vi "operate.vi"(10 "symbol":string[](array[string]), 11 "Element":string[](array[string])) -> (2 "Value":dbl, 3 "Result":string)   [LabVIEW 2020]
uses:
  <vilib>/Analysis/NI_AALBase.lvlib
  <vilib>/Analysis/baseanly.llb/Mean (DBL).vi
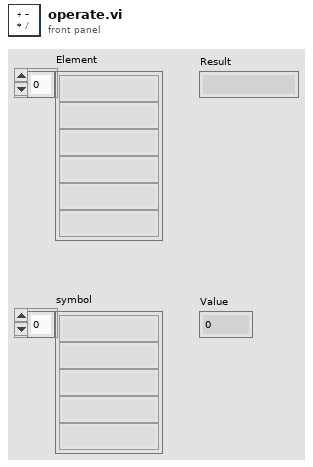
[diagram p1: front panel]
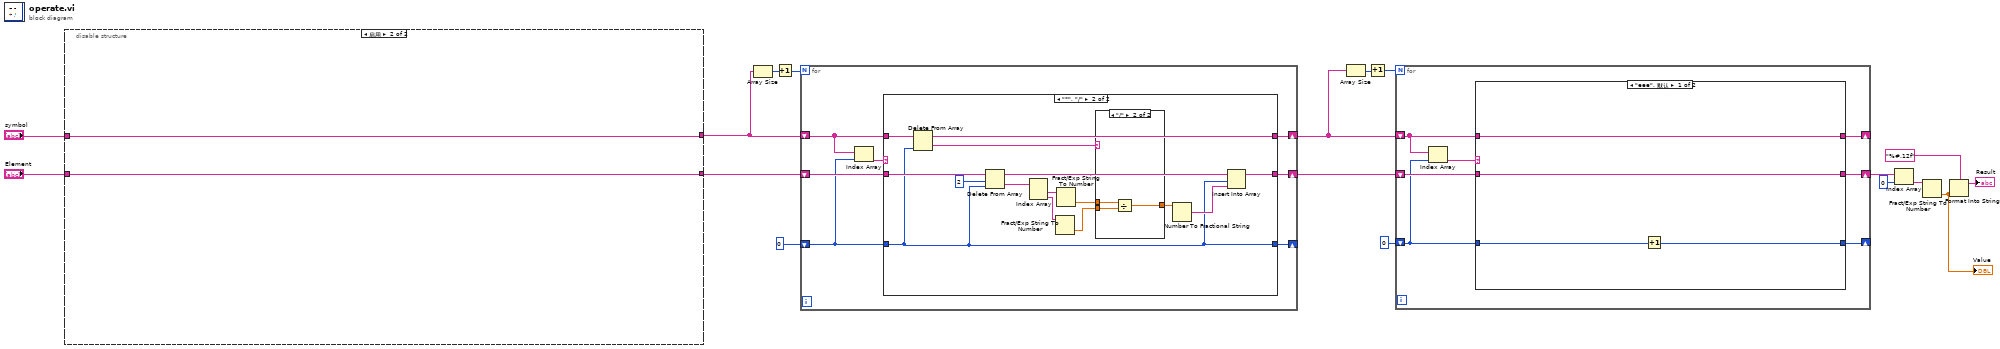
[diagram p0: block diagram]
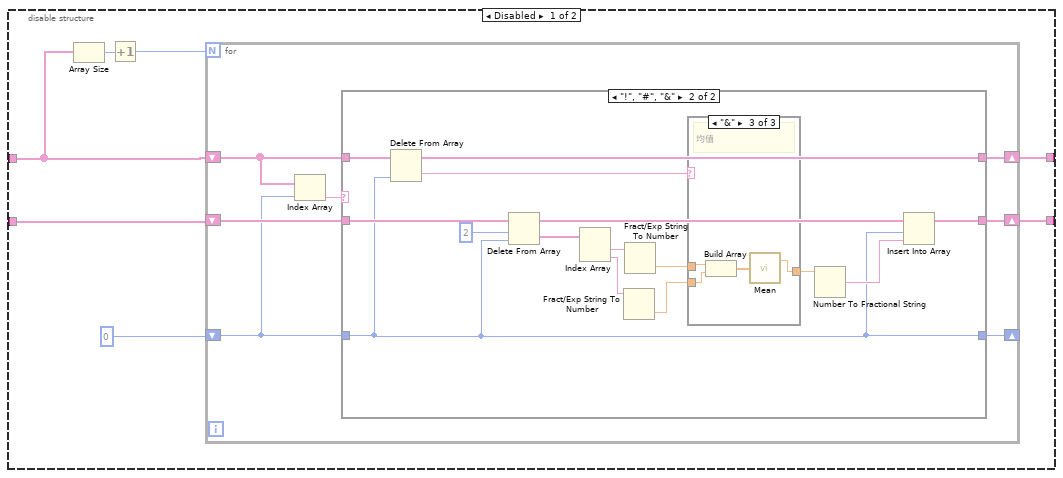
[diagram p2: hidden frame]
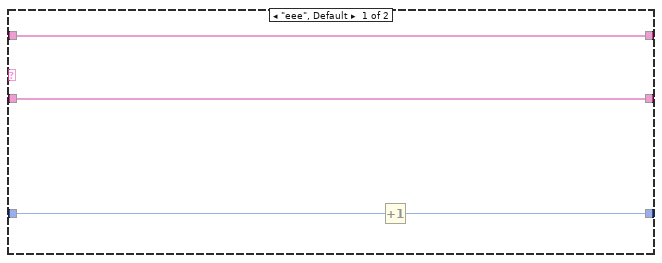
[diagram p3: hidden frame]
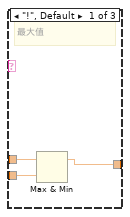
[diagram p4: hidden frame]
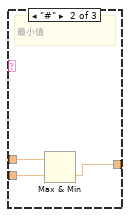
[diagram p5: hidden frame]
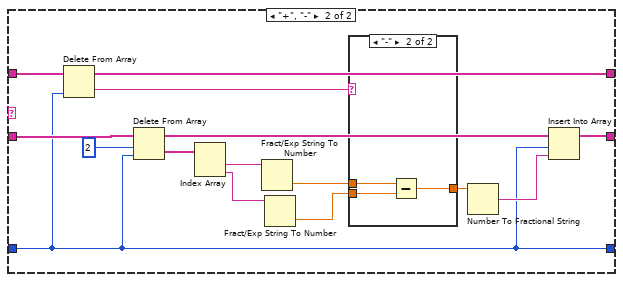
[diagram p6: hidden frame]
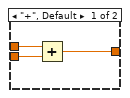
[diagram p7: hidden frame]
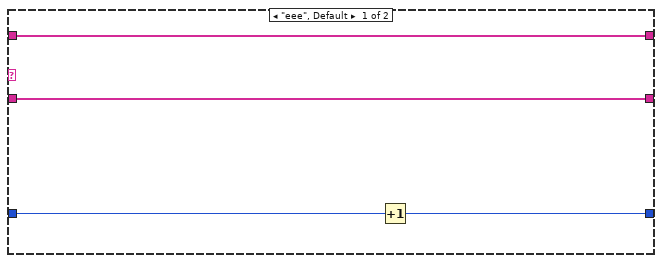
[diagram p8: hidden frame]
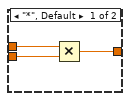
[diagram p9: hidden frame]
diagram:
  n1 = disable-structure shown="启用" {
    disable-tunnel: "symbol" -> [w24 w63]
    disable-tunnel: [w23 w63] -> w5
    disable-tunnel: "Element" -> [w21 w62]
    disable-tunnel: [w20 w62] -> w2
    frame Disabled {
      n2 = Array Size(array=w24) -> (size(s)=w25:i32)
      n3 = Increment(x=w25) -> (x+1=w22:i32)
      n4 = for {
        N: w22 -> [_]
        shift-right: [w31] -> w20
        shift-left: w21 -> [w32]
        shift-right: [w28] -> w23
        shift-left: w24 -> [w29]
        shift-right: [w26] -> _
        shift-left: 0 -> [w27]
        n5 = Index Array(array=w29, index=w27) -> (element=w30:string)
        n6 = case shown="\"!\", \"#\", \"&\"" w30 {
          tunnel: w32 -> [w36 w48]
          tunnel: w27 -> [w33 w40]
          tunnel: [w36 w43] -> w31
          tunnel: w29 -> [w35 w42]
          tunnel: [w35 w41] -> w28
          tunnel: [w34 w40] -> w26
          frame "eee", Default {
            n7 = Increment(x=w33) -> (x+1=w34:i32)
          }
          frame "!", "#", "&" {
            n8 = Delete From Array(array=w42, index=w40) -> (deleted portion=w39:string, array with subset deleted=w41:string[])  [unwired: 1 in]
            n9 = Delete From Array(array=w48, length=2 ("长度"), index=w40) -> (deleted portion=w37:string[], array with subset deleted=w46:string[])
            n10 = Index Array(array=w37) -> (element #1=w51:string, element #2=w38:string)  [unwired: 2 in]
            n11 = Fract/Exp String To Number(string=w38) -> (number=w49:dbl)  [unwired: 3 in, 1 out]
            n12 = Fract/Exp String To Number(string=w51) -> (number=w50:dbl)  [unwired: 3 in, 1 out]
            n13 = case shown="\"&\"" w39 {
              tunnel: w50 -> [w54 w57 w59]
              tunnel: w49 -> [w53 w56 w61]
              tunnel: [w52 w55 w58] -> w45
              frame "!", Default {
                # "最大值"
                n14 = Max & Min(x=w54, y=w53) -> (max(x,y)=w52:dbl)  [unwired: 1 out]
              }
              frame "#" {
                # "最小值"
                n15 = Max & Min(x=w57, y=w56) -> (min(x,y)=w55:dbl)  [unwired: 1 out]
              }
              frame "&" {
                # "均值"
                n16 = Build Array(w59, w61) -> (w60:dbl[])
                n17 = call-poly <vilib>:"Mean.vi"("X"=w60) -> ("mean"=w58:dbl)  [unwired: 1 out]
              }
            }
            n18 = Number To Fractional String(number=w45) -> (F-format string=w44:string)  [unwired: 3 in]
            n19 = Insert Into Array(array=w46, index=w40, new element=w44) -> (w43:string[])
          }
        }
      }
    }
    frame Enabled {
    }
  }
  n20 = Array Size(array=w5) -> (size(s)=w7:i32)
  n21 = Increment(x=w7) -> (x+1=w4:i32)
  n22 = for {
    N: w4 -> [_]
    shift-right: [w69] -> w14
    shift-left: w2 -> [w70]
    shift-right: [w66] -> w15
    shift-left: w5 -> [w67]
    shift-right: [w64] -> _
    shift-left: 0 -> [w65]
    n23 = Index Array(array=w67, index=w65) -> (element=w68:string)
    n24 = case shown="\"*\", \"/\"" w68 {
      tunnel: w70 -> [w74 w86]
      tunnel: w65 -> [w71 w78]
      tunnel: [w74 w81] -> w69
      tunnel: w67 -> [w73 w80]
      tunnel: [w73 w79] -> w66
      tunnel: [w72 w78] -> w64
      frame "eee", Default {
        n25 = Increment(x=w71) -> (x+1=w72:i32)
      }
      frame "*", "/" {
        n26 = Delete From Array(array=w80, index=w78) -> (deleted portion=w77:string, array with subset deleted=w79:string[])  [unwired: 1 in]
        n27 = Delete From Array(array=w86, length=2 ("长度"), index=w78) -> (deleted portion=w75:string[], array with subset deleted=w84:string[])
        n28 = Index Array(array=w75) -> (element #1=w89:string, element #2=w76:string)  [unwired: 2 in]
        n29 = Fract/Exp String To Number(string=w76) -> (number=w87:dbl)  [unwired: 3 in, 1 out]
        n30 = Fract/Exp String To Number(string=w89) -> (number=w88:dbl)  [unwired: 3 in, 1 out]
        n31 = case shown="\"/\"" w77 {
          tunnel: w88 -> [w92 w95]
          tunnel: w87 -> [w91 w94]
          tunnel: [w90 w93] -> w83
          frame "*", Default {
            n32 = Multiply(x=w92, y=w91) -> (x*y=w90:dbl)
          }
          frame "/" {
            n33 = Divide(x=w95, y=w94) -> (x/y=w93:dbl)
          }
        }
        n34 = Number To Fractional String(number=w83) -> (F-format string=w82:string)  [unwired: 3 in]
        n35 = Insert Into Array(array=w84, index=w78, new element=w82) -> (w81:string[])
      }
    }
  }
  n36 = Array Size(array=w15) -> (size(s)=w16:i32)
  n37 = Increment(x=w16) -> (x+1=w17:i32)
  n38 = for {
    N: w17 -> [_]
    shift-right: [w101] -> w13
    shift-left: w14 -> [w102]
    shift-right: [w98] -> _
    shift-left: w15 -> [w99]
    shift-right: [w96] -> _
    shift-left: 0 -> [w97]
    n39 = Index Array(array=w99, index=w97) -> (element=w100:string)
    n40 = case shown="\"eee\", 默认" w100 {
      tunnel: w102 -> [w106 w118]
      tunnel: w97 -> [w103 w109]
      tunnel: [w106 w113] -> w101
      tunnel: w99 -> [w105 w112]
      tunnel: [w105 w111] -> w98
      tunnel: [w104 w109] -> w96
      frame "eee", Default {
        n41 = Increment(x=w103) -> (x+1=w104:i32)
      }
      frame "+", "-" {
        n42 = Delete From Array(array=w112, index=w109) -> (deleted portion=w110:string, array with subset deleted=w111:string[])  [unwired: 1 in]
        n43 = Delete From Array(array=w118, length=2 ("长度"), index=w109) -> (deleted portion=w108:string[], array with subset deleted=w116:string[])
        n44 = Index Array(array=w108) -> (element #1=w121:string, element #2=w107:string)  [unwired: 2 in]
        n45 = Fract/Exp String To Number(string=w121) -> (number=w120:dbl)  [unwired: 3 in, 1 out]
        n46 = Fract/Exp String To Number(string=w107) -> (number=w119:dbl)  [unwired: 3 in, 1 out]
        n47 = case shown="\"-\"" w110 {
          tunnel: w120 -> [w124 w127]
          tunnel: w119 -> [w123 w126]
          tunnel: [w122 w125] -> w115
          frame "+", Default {
            n48 = Add(x=w124, y=w123) -> (x+y=w122:dbl)
          }
          frame "-" {
            n49 = Subtract(x=w127, y=w126) -> (x-y=w125:dbl)
          }
        }
        n50 = Number To Fractional String(number=w115) -> (F-format string=w114:string)  [unwired: 3 in]
        n51 = Insert Into Array(array=w116, index=w109, new element=w114) -> (w113:string[])
      }
    }
  }
  n52 = Index Array(array=w13, index=0 ("索引")) -> (element=w8:string)
  n53 = Fract/Exp String To Number(string=w8) -> (number=w10:dbl)  [unwired: 3 in, 1 out]
  "Value" <- w10
  n54 = Format Into String(format string="%#.12f" ("格式字符串"), w10) -> (resulting string=→"Result":string)  [unwired: 2 in, 1 out]
